vi "DS Functions.vi"() -> ()   [LabVIEW 2026]
uses:
  vi.lib/Rock Robotics/WPI/Joystick/WPI_JoystickDeviceEnum.ctl
  vi.lib/MRC/MrcLib/MrcLib.lvlib
panel:
  out "Axes":dbl[](array[numeric])
  out "POVs":u8[](array[numeric])
  out "Info":T1
  in  "rumble":cluster{"Left":sgl, "Right":sgl}
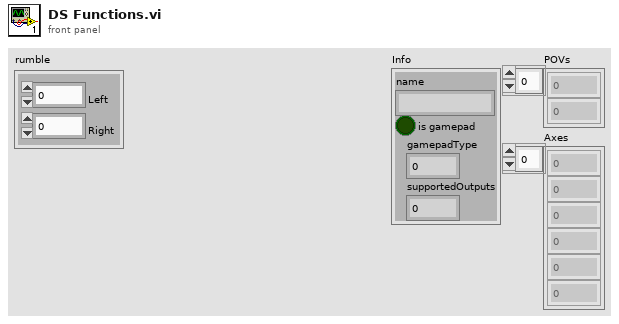
[diagram p1: front panel]
types:
  T1 = cluster{"name":string, "is gamepad":bool, "gamepadType":u8, "supportedOutputs":u8}
  T2 = typedef "WPI_JoystickDeviceEnum.ctl" = enum16{"USB 0", "USB 1", "USB 2", "USB 3", "USB 4", "USB 5"}
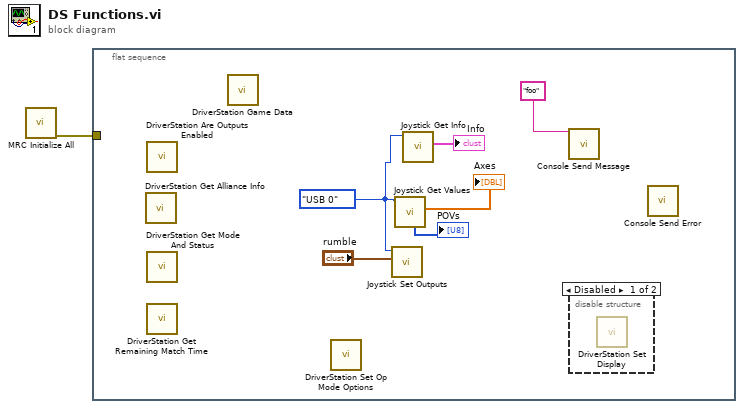
[diagram p0: block diagram]
diagram:
  n1 = call "MRC Initialize All.vi"() -> ("error out"=w1:errorcluster)  [unwired: 11 in]
  n2 = flat-sequence {
    tunnel: w1 -> [_]
    frame #0 {
      w7 = WPI_JoystickDeviceEnum."USB 0" ("Joystick")
      n3 = call "DriverStation Get Alliance Info.vi"() -> ()  [unwired: 7 in, 5 out]
      n4 = call "DriverStation Are Outputs Enabled.vi"() -> ()  [unwired: 10 in, 2 out]
      n5 = call "DriverStation Get Mode And Status.vi"() -> ()  [unwired: 8 in, 4 out]
      n6 = call "DriverStation Get Remaining Match Time.vi"() -> ()  [unwired: 9 in, 3 out]
      n7 = call "DriverStation Game Data.vi"() -> ()  [unwired: 11 in, 1 out]
      n8 = call "DriverStation Set Op Mode Options.vi"() -> ()  [unwired: 11 in, 1 out]
      n9 = call "Joystick Set Outputs.vi"("rumble"="rumble", "Joystick"=w7) -> ()  [unwired: 8 in, 2 out]
      n10 = call "Joystick Get Values.vi"("Joystick"=w7) -> ("Axes"=→"Axes":dbl[], "POVs"=→"POVs":u8[])  [unwired: 5 in, 4 out]
      n11 = call "Joystick Get Info.vi"("Joystick"=w7) -> ("Info"=→"Info":T1)  [unwired: 8 in, 2 out]
      n12 = call "Console Send Message.vi"("Message"="foo") -> ()  [unwired: 14 in, 1 out]
      n13 = disable-structure shown="Disabled" {
        frame Disabled {
          n14 = call "DriverStation Set Display.vi"() -> ()  [unwired: 11 in, 1 out]
        }
        frame Enabled {
        }
      }
      n15 = call "Console Send Error.vi"() -> ()  [unwired: 15 in, 1 out]
    }
  }
